vi "Write Depth Values.vi"(8 "error in (no error)":errorcluster, 10 "Depth Values":dbl[][](array[numeric]), 11 "Video Frame in":refnum<class "Video Frame.lvclass">) -> (0 "error out":errorcluster, 3 "Video Frame out":refnum<class "Video Frame.lvclass">)   [LabVIEW 2018, in "Video Frame.lvclass"]
uses:
  Video Frame.lvclass
  Video Frame.lvclass/Video Frame.ctl
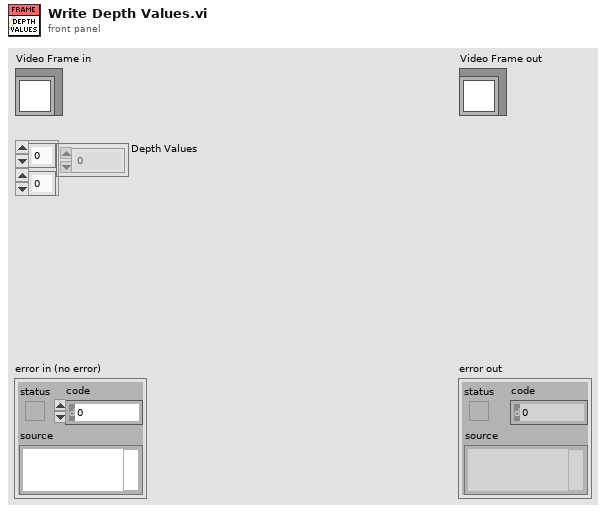
[diagram p1: front panel]
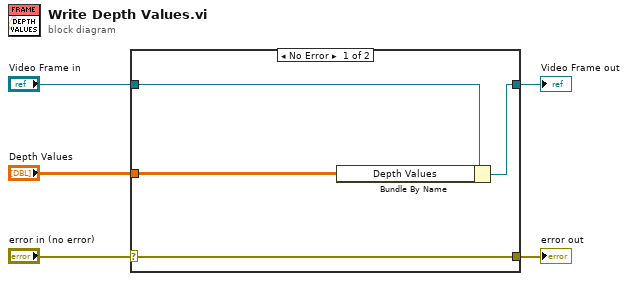
[diagram p0: block diagram]
diagram:
  n1 = case shown="No Error" "error in (no error)" {
    selector: "error in (no error)" -> [w9 w10]
    tunnel: [w9 w10] -> w4
    tunnel: [w7 w11] -> w2
    tunnel: "Video Frame in" -> [w8 w11]
    tunnel: "Depth Values" -> [w6 _]
    frame No Error {
      n2 = Bundle By Name(cluster=w8, "Depth Values"=w6) -> (w7:refnum<class "Video Frame.lvclass">)
    }
    frame Error {
    }
  }
  "error out" <- w4
  "Video Frame out" <- w2
